vi "Get Encoder Data.vi"(9 "Reset Position":bool, 10 "error in":errorcluster, 11 "FPGA_MAIN ref in":T1) -> (0 "Right Dist. Travelled (Cm)":dbl, 1 "Left Dist. Travelled (Cm)":dbl, 2 "error out":errorcluster, 3 "FPGA_MAIN ref out":T1, 4 "Right Acceleration (rps/s)":dbl, 5 "Right Velocity (RPM)":dbl, 6 "Left Acceleration (rps/s)":dbl, 7 "Left Velocity (RPM)":dbl, 8 "Encoders Zeroed?":bool)   [LabVIEW 2009]
doc: "Real Time Host vi for Quadrature Encoder Velocity and Acceleration Estimation using CompactRIO.\n\nThis application is designed to work with an R-Series expansion setup using FPGA-7811R and a CompactRIO cRIO-9411 digital input module installed in slot 1 of the expansion chassis.\n\nBefore Executing the vi:\n1. Select the FPGA Resource in the VISA Resource Name Control\n2. Specify a Fixed Time Interval for Velocity and Acceleration Estimation\n3. Specify the Pulses/revolution for the Quadrature Encoder\n4. Run the vi"
uses:
  TypeDefs/Sensor TypeDefs/FPGA Main ref.ctl
  <vilib>/rvi/interface/nirviReadWriteControl/nirviReadWriteControl.xnode
  FPGA Bitfiles/Q_IGVC_2010.lvproj_FPGA Target_FPGA_MAIN.vi.lvbitx
  <vilib>/Utility/error.llb/Error Cluster From Error Code.vi
  <vilib>/rvi/errors/niLvFpgaAdjustHostInterfaceError.vi
  <vilib>/rvi/interface/common/niFpgaNodeNameForErrorReporting.ctl
  <vilib>/rvi/errors/niLvFpgaWhatHappensToTopLevelVI.ctl
  NiRioSrv.dll
panel:
  out "Left Position (Counts)":i32
  out "Right Position (Counts)":i32
  in  "Pulses/Revolution":i32=2000
  in  "Fixed Time \nInterval (uSec)":u32=1000
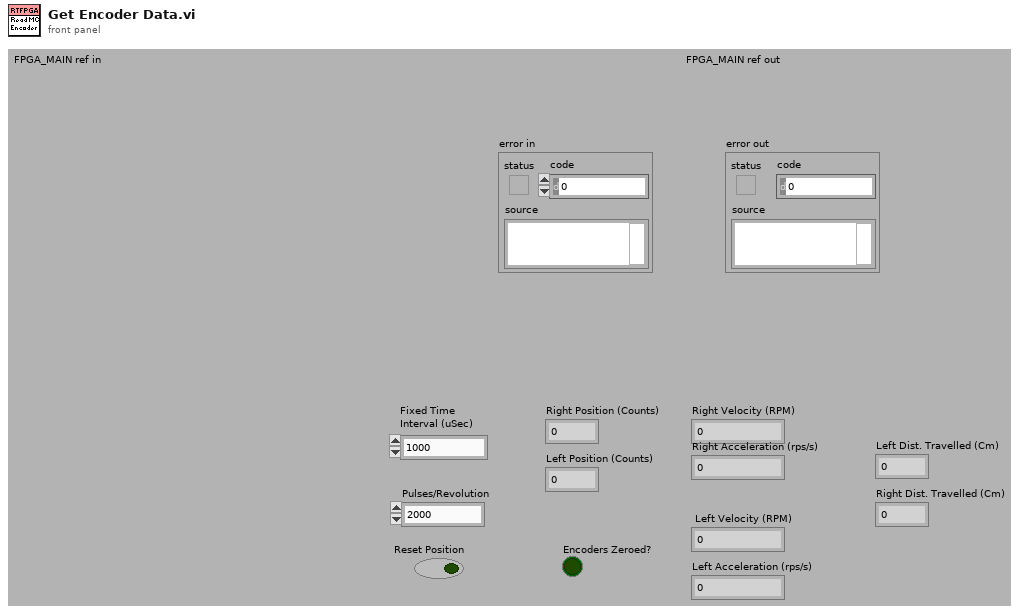
[diagram p1: front panel]
types:
  T1 = typedef "FPGA Main ref.ctl" = refnum<k20>
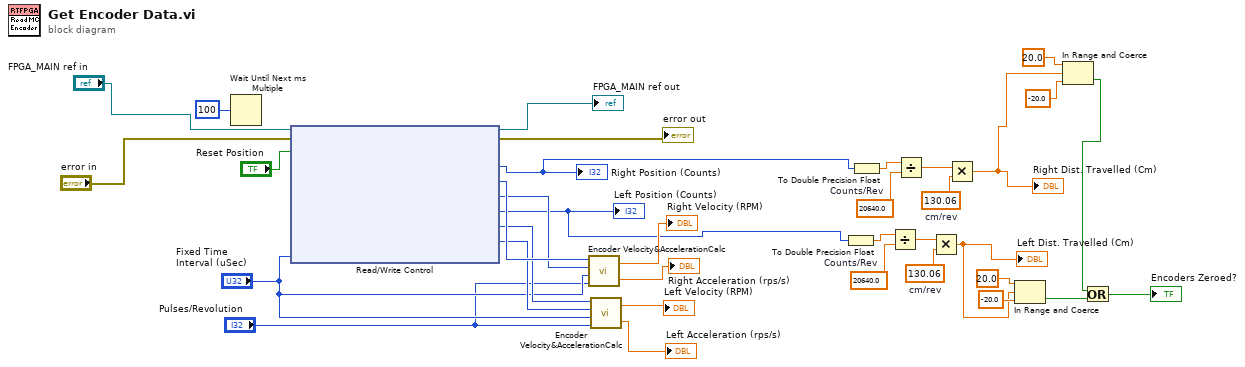
[diagram p0: block diagram]
diagram:
  w14 = 130.06  # cm/rev
  w15 = 130.06  # cm/rev
  w18 = 20640.0  # Counts/Rev
  w21 = 20640.0  # Counts/Rev
  n1 = Wait Until Next ms Multiple(millisecond multiple=u32 100) -> ()  [unwired: 1 out]
  n2 = xnode "Read/Write Control"("FPGA VI Reference In"="FPGA_MAIN ref in", "error in"="error in", "Position Reset"="Reset Position", "Velocity Interval (uSec)"="Fixed Time \nInterval (uSec)") -> ("FPGA VI Reference Out"=→"FPGA_MAIN ref out":T1, "error out"=→"error out":errorcluster, "Right Position (Counts)"=w20:i32, "Right Velocity (Counts/Interval)"=w33:i32, "Right Acceleration (Counts/Interval)"=w31:i32, "Left Position (Counts)"=w17:i32, "Left Velocity (Counts/Interval)"=w30:i32, "Left Acceleration (Counts/Interval)"=w29:i32)
  "Right Position (Counts)" <- w20
  "Left Position (Counts)" <- w17
  n3 = call "Encoder Velocity&AccelerationCalc.vi"("Pulses/Revolution"="Pulses/Revolution", "Fixed Time \nInterval (uSec)"="Fixed Time \nInterval (uSec)", "Acceleration (Counts/Interval)"=w31, "Velocity (Counts/Interval)"=w33) -> ("Acceleration (rps/s)"=→"Right Acceleration (rps/s)":dbl, "Velocity (RPM)"=→"Right Velocity (RPM)":dbl)
  n4 = call "Encoder Velocity&AccelerationCalc.vi"("Pulses/Revolution"="Pulses/Revolution", "Fixed Time \nInterval (uSec)"="Fixed Time \nInterval (uSec)", "Acceleration (Counts/Interval)"=w29, "Velocity (Counts/Interval)"=w30) -> ("Acceleration (rps/s)"=→"Left Acceleration (rps/s)":dbl, "Velocity (RPM)"=→"Left Velocity (RPM)":dbl)
  n5 = To Double Precision Float(number=w17) -> (double precision float=w19:dbl)
  n6 = To Double Precision Float(number=w20) -> (double precision float=w22:dbl)
  n7 = Divide(x=w19, y=w18) -> (x/y=w13:dbl)
  n8 = Divide(x=w22, y=w21) -> (x/y=w16:dbl)
  n9 = Multiply(x=w13, y=w14) -> (x*y=w3:dbl)
  "Left Dist. Travelled (Cm)" <- w3
  n10 = Multiply(x=w16, y=w15) -> (x*y=w9:dbl)
  "Right Dist. Travelled (Cm)" <- w9
  n11 = In Range and Coerce(upper limit=20.0, x=w3, lower limit=-20.0) -> (In Range?=w2:bool)  [unwired: 1 out]
  n12 = In Range and Coerce(upper limit=20.0, x=w9, lower limit=-20.0) -> (In Range?=w8:bool)  [unwired: 1 out]
  n13 = Or(x=w8, y=w2) -> (x .or. y?=→"Encoders Zeroed?":bool)
